vi "C4Buf_getFeatureType.vi"(0 "c4buf in":refnum<k24>, 7 "name in":string, 11 "error in":errorcluster) -> (4 "c4buf out":refnum<k24>, 8 "featureType out":i64(ring) items=["UNKNOWN", "INTEGER", "FLOAT", "STRING", "ENUMERATION", "COMMAND", "BOOLEAN"], 15 "error out":errorcluster)   [LabVIEW 2015, in "libC4HdlLV.lvlib"]
uses:
  libC4HdlLV.lvlib
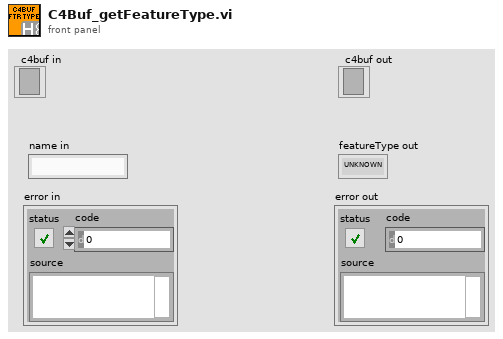
[diagram p1: front panel]
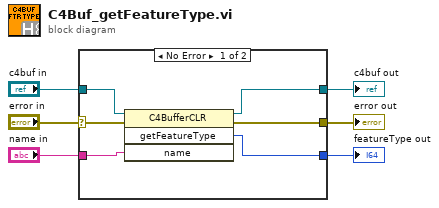
[diagram p0: block diagram]
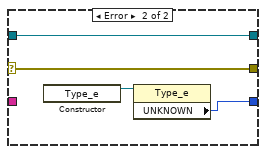
[diagram p2: hidden frame]
diagram:
  n1 = case shown="No Error" "error in" {
    selector: "error in" -> [w9 w16]
    tunnel: [w8 w16] -> w5
    tunnel: "c4buf in" -> [w12 w15]
    tunnel: [w10 w15] -> w4
    tunnel: [w11 w14] -> w2
    tunnel: "name in" -> [w7 _]
    frame No Error {
      n2 = invoke class="C4BufferCLR" method="getFeatureType"(reference=w12, error in=w9, "name"=w7) -> (reference out=w10:refnum<k24>, error out=w8:errorcluster, "getFeatureType"=w11:i64)  [unwired: 1 in, 1 out]
    }
    frame Error {
      n3 = constructor class="Type_e"() -> (reference out=w13:refnum<k24>)  [unwired: 3 in, 2 out]
      n4 = property class="Type_e"(reference=w13) -> ("UNKNOWN"=w14:i64)  [unwired: 1 in, 2 out]
    }
  }
  "error out" <- w5
  "c4buf out" <- w4
  "featureType out" <- w2
